vi "Upsample.vi"   [LabVIEW 2010, in "NI_AALPro.lvlib"]
doc: "Inserts zeros in input sequence <B>X</B> by <B>upsampling factor</B>. Wire data to the <B>X</B> input to determine the polymorphic instance to use or manually select the instance."
uses:
  NI_AALPro.lvlib
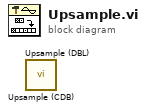
[diagram p0: block diagram]
diagram:
  n1 = call "Upsample (CDB).vi"() -> ()  [unwired: 10 in, 2 out]
  n2 = call "Upsample (DBL).vi"() -> ()  [unwired: 10 in, 2 out]
